vi "Gather Statistics.vi"(10 "JSON Object":refnum<class "JSON Object.lvclass">, 11 "JSON Value In":refnum<class "JSON Value.lvclass">) -> (3 "JSON Statistic or Object":refnum<class "JSON Value.lvclass">)   [LabVIEW 2020, in "Library Commun.lvlib" / "JSON Object.lvclass"]
uses:
  JSON Object.lvclass
  JSON Value/JSON Value.lvclass
  C:/Users/ngarcin/OneDrive - Altyor/Standard TB/Class/JSON API/JSON Value/JSON Value.lvclass
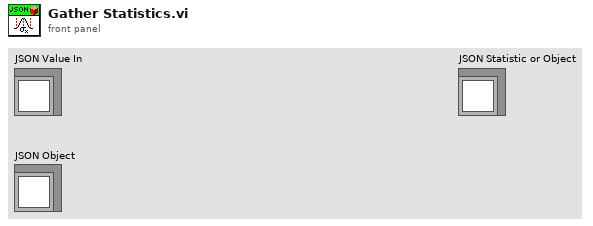
[diagram p1: front panel]
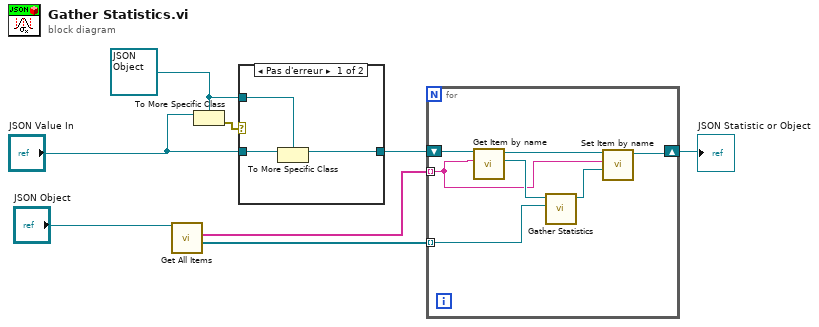
[diagram p0: block diagram]
diagram:
  w5 = refnum<class "JSON Object.lvclass"> refnum ("JSON Object")
  n1 = call-dynamic "Get All Items.vi"("JSON Object in"="JSON Object") -> ("Values"=w2:refnum<class "JSON Value.lvclass">[], "Item Names"=w3:string[])  [unwired: 7 in, 2 out]
  n2 = To More Specific Class(target class=w5, reference="JSON Value In") -> (error out=w7:errorcluster)  [unwired: 1 in, 1 out]
  n3 = case shown="Pas d'erreur" w7 {
    tunnel: "JSON Value In" -> [w11 _]
    tunnel: w5 -> [w10 _]
    tunnel: [w9 _] -> w4
    frame No Error {
      n4 = To More Specific Class(target class=w10, reference=w11) -> (specific class reference=w9:refnum<class "JSON Object.lvclass">)  [unwired: 1 in, 1 out]
    }
    frame Error {
    }
  }
  n5 = for {
    shift-right: [w14] -> w1
    shift-left: w4 -> [w18]
    tunnel: w3 -> [w13] mode=indexing
    tunnel: w2 -> [w16] mode=indexing
    n6 = call-dynamic "Get Item by name.vi"("name"=w13, "JSON Object in"=w18) -> ("Value"=w17:refnum<class "JSON Value.lvclass">, "JSON Object out"=w15:refnum<class "JSON Object.lvclass">)  [unwired: 6 in, 2 out]
    n7 = call-dynamic "Gather Statistics.vi"("JSON Value"=w16, "Statistics in"=w17) -> ("Statistics out"=w12:refnum<class "JSON Value.lvclass">)  [unwired: 9 in]
    n8 = call-dynamic "Set Item by name.vi"("Value"=w12, "name"=w13, "JSON Object in"=w15) -> ("JSON Object out"=w14:refnum<class "JSON Object.lvclass">)  [unwired: 6 in, 2 out]
  }
  "JSON Statistic or Object" <- w1
